vi "Get Size.vi"   [LabVIEW 2019, in "xy_utilities.lvlib"]
uses:
  xy_utilities.lvlib
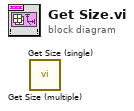
[diagram p0: block diagram]
diagram:
  n1 = call "Get Size (multiple).vi"() -> ()  [unwired: 8 in, 4 out]
  n2 = call "Get Size (single).vi"() -> ()  [unwired: 8 in, 4 out]
